vi "Parse Parameter.vi"(6 "error text in":string, 8 "error in":errorcluster, 11 "node in":refnum<k20>) -> (0 "error out":errorcluster, 3 "parametesrs":T1[](array[typedef]))   [LabVIEW 2024, in "ARINC 429 Import.lvlib"]
uses:
  ARINC 429 Import.lvlib
  Shared/VS Channel Definition for Parameter.ctl
  Shared/Parameter Definition.ctl
  <vilib>/NI/NI VeriStand Encoding and Decoding/Encoding.ctl
  Read Tag Element (String).vi
  Read Tag Element (DBL).vi
  Read Tag Element (I32).vi
  Read Tag Element (Boolean).vi
  <vilib>/NI/NI VeriStand Encoding and Decoding/Encoding and Decoding.lvlib
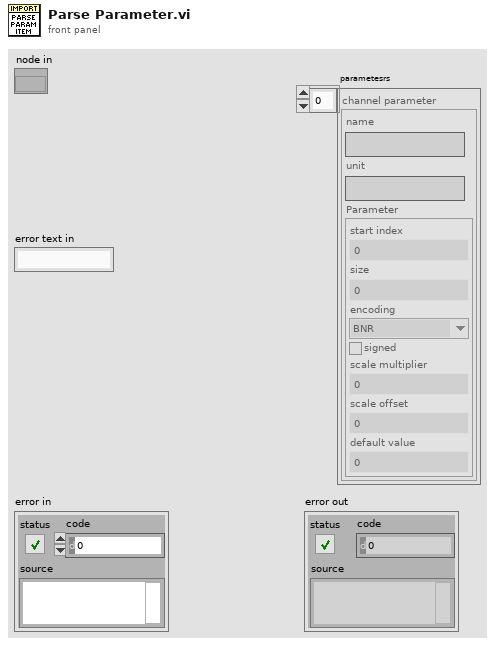
[diagram p1: front panel]
types:
  T1 = typedef "VS Channel Definition for Parameter.ctl" = cluster{"name":string, "unit":string, "Parameter":T2}
  T2 = typedef "Parameter Definition.ctl" = cluster{"start index":i32, "size":i32, "encoding":T3, "signed":bool, "scale multiplier":dbl, "scale offset":dbl, "default value":dbl}
  T3 = typedef "Encoding and Decoding.lvlib/Encoding.ctl" = enum16{"BNR", "BCD", "Discrete"}
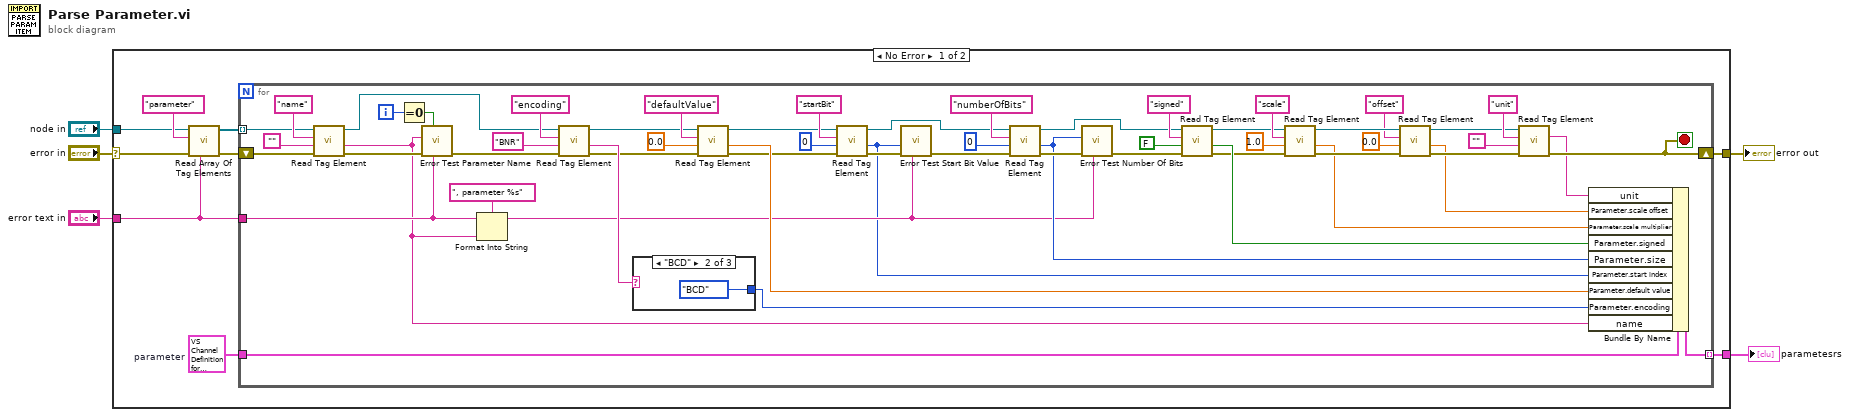
[diagram p0: block diagram]
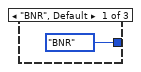
[diagram p2: hidden frame]
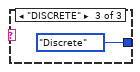
[diagram p3: hidden frame]
diagram:
  n1 = case shown="No Error" "error in" {
    selector: "error in" -> [w9 w75]
    tunnel: "node in" -> [w11 _]
    tunnel: [w10 w75] -> w4
    tunnel: "error text in" -> [w8 _]
    tunnel: [w7 _] -> w1
    frame No Error {
      w6 = T1 {"name"="", "unit"="", "Parameter"={"start index"=0, "size"=8, "encoding"=enum."BCD", "signed"=FALSE, "scale multiplier"=1.0, "scale offset"=0.0, "default value"=0.0}}  # parameter
      n2 = call "Read Array Of Tag Elements.vi"("error text in"=w8, "error in"=w9, "tag name"="parameter" ("Tag Name"), "node in"=w11) -> ("error out"=w13:errorcluster, "array of elements"=w12:refnum<k20>[])  [unwired: 6 in]
      n3 = for {
        shift-right: [w31] -> w10
        shift-left: w13 -> [w69]
        tunnel: w12 -> [w37] mode=indexing
        tunnel: w8 -> [w22]
        tunnel: [w16] -> w7 mode=indexing
        tunnel: w6 -> [w15]
        i -> [w25]
        stop <- w31 stop-if-true
        n4 = call-poly "Read Tag Element.vi"("error in"=w69, "default"="", "Tag Name"="name", "node in"=w37) -> ("error out"=w27:errorcluster, "value"=w20:string, "node out"=w23:refnum<k20>)  [unwired: 5 in]
        n5 = Equal To 0?(x=w25) -> (x = 0?=w24:bool)
        n6 = call "Error Test Parameter Name.vi"("error text in"=w22, "reset (F)"=w24, "error in"=w27, "parameter name"=w20) -> ("error out"=w26:errorcluster)  [unwired: 7 in]
        n7 = Format Into String(format string=", parameter %s", initial string=w22, w20) -> (resulting string=w29:string)  [unwired: 1 in, 1 out]
        n8 = call-poly "Read Tag Element.vi"("error in"=w26, "default"="BNR", "Tag Name"="encoding", "node in"=w23) -> ("error out"=w62:errorcluster, "value"=w66:string, "node out"=w63:refnum<k20>)  [unwired: 5 in]
        n9 = case shown="\"BCD\"" w66 {
          tunnel: [Encoding."BNR" ("Encoding Type") Encoding."BCD" ("Encoding Type") Encoding."Discrete" ("Encoding Type")] -> w21
          frame "BNR", Default {
          }
          frame "BCD" {
          }
          frame "DISCRETE" {
          }
        }
        n10 = call-poly "Read Tag Element.vi"("error in"=w62, "default"=0.0, "Tag Name"="defaultValue", "node in"=w63) -> ("error out"=w54:errorcluster, "value"=w61:dbl, "node out"=w58:refnum<k20>)  [unwired: 5 in]
        n11 = call-poly "Read Tag Element.vi"("error in"=w54, "default"=0, "Tag Name"="startBit", "node in"=w58) -> ("error out"=w36:errorcluster, "value"=w28:i32, "node out"=w55:refnum<k20>)  [unwired: 5 in]
        n12 = call "Error Test Start Bit Value.vi"("error text in"=w29, "error in"=w36, "start bit"=w28) -> ("error out"=w35:errorcluster)  [unwired: 8 in]
        n13 = call-poly "Read Tag Element.vi"("error in"=w35, "default"=0, "Tag Name"="numberOfBits", "node in"=w55) -> ("error out"=w34:errorcluster, "value"=w32:i32, "node out"=w51:refnum<k20>)  [unwired: 5 in]
        n14 = call "Error Test Number Of Bits.vi"("error text in"=w29, "error in"=w34, "number of bits"=w32) -> ("error out"=w33:errorcluster)  [unwired: 8 in]
        n15 = call-poly "Read Tag Element.vi"("error in"=w33, "default"=FALSE, "Tag Name"="signed", "node in"=w51) -> ("error out"=w42:errorcluster, "value"=w50:bool, "node out"=w43:refnum<k20>)  [unwired: 5 in]
        n16 = call-poly "Read Tag Element.vi"("error in"=w42, "default"=1.0, "Tag Name"="scale", "node in"=w43) -> ("error out"=w49:errorcluster, "value"=w17:dbl, "node out"=w48:refnum<k20>)  [unwired: 5 in]
        n17 = call-poly "Read Tag Element.vi"("error in"=w49, "default"=0.0, "Tag Name"="offset", "node in"=w48) -> ("error out"=w38:errorcluster, "value"=w18:dbl, "node out"=w39:refnum<k20>)  [unwired: 5 in]
        n18 = call-poly "Read Tag Element.vi"("error in"=w38, "default"="", "Tag Name"="unit", "node in"=w39) -> ("error out"=w31:errorcluster, "value"=w19:string)  [unwired: 5 in, 1 out]
        n19 = Bundle By Name(cluster=w15, "unit"=w19, "Parameter.scale offset"=w18, "Parameter.scale multiplier"=w17, "Parameter.signed"=w50, "Parameter.size"=w32, "Parameter.start index"=w28, "Parameter.default value"=w61, "Parameter.encoding"=w21, "name"=w20) -> (w16:T1)
      }
    }
    frame Error {
    }
  }
  "parametesrs" <- w1
  "error out" <- w4
